vi "Desktop Execution Node - Test Tachometer and Fan Speed IP.vi"() -> ()   [LabVIEW 2014]
uses:
  <vilib>/rvi/DesktopExecutionNode/Execution/niFpgaDEN_Execute.vi
  <vilib>/rvi/DesktopExecutionNode/DesktopExecutionNode.xnode
panel:
  in  "stop":bool
  out "Fan Speed (RPM) Chart":sgl(graph)
  out "Simulated Tachometer Signal":dbl[](graph)
  out "Iteration":i32
  in  "Tach data filename":path=path "Tach - 3000 RPM.tdms"
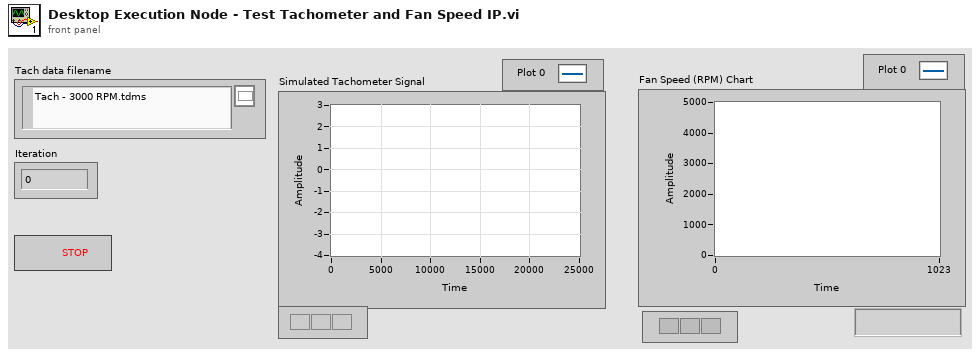
[diagram p1: front panel]
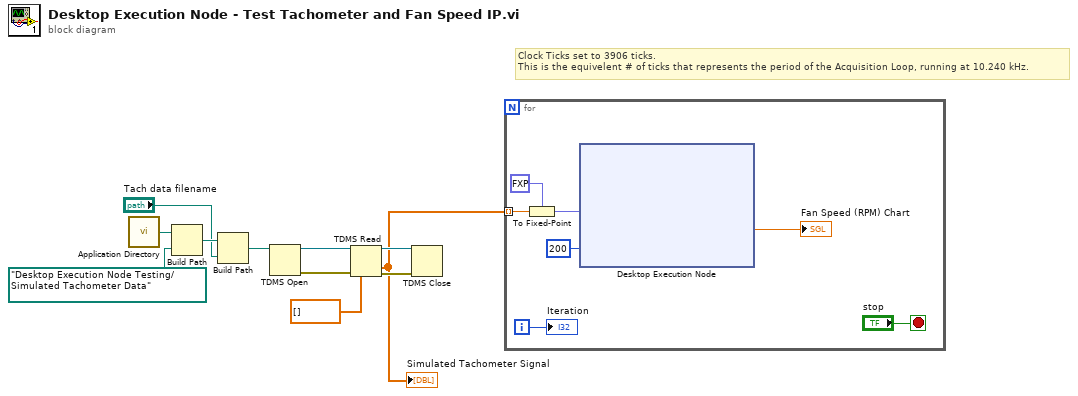
[diagram p0: block diagram]
diagram:
  # "Clock Ticks set to 3906 ticks.\nThis is the equivelent # of ticks that represents the period of the Acquisition Loop, running at 10.240 kHz."
  n1 = call <vilib>:"Application Directory.vi"() -> ("Application Directory"=w5:path)
  n2 = Build Path(base path=w5, name or relative path=path "Desktop Execution Node Testing/Simulated Tachometer Data" ("Application Directory")) -> (appended path=w3:path)
  n3 = Build Path(base path=w3, name or relative path="Tach data filename") -> (appended path=w1:path)
  n4 = TDMS Open(11:w1) -> (0:w10:errorcluster, 3:w11:refnum<k34>)  [unwired: 6 in]
  n5 = TDMS Read(0:w11, 11:w10, 12:dbl[] []) -> (4:w7:refnum<k34>, 10:w6:dbl[], 15:w8:errorcluster)  [unwired: 5 in, 3 out]
  "Simulated Tachometer Signal" <- w6
  n6 = TDMS Close(8:w8, 11:w7) -> ()  [unwired: 2 out]
  n7 = for {
    tunnel: w6 -> [w18] mode=indexing
    i -> [w15]
    stop <- "stop" stop-if-true
    n8 = To Fixed-Point(fixed-point type=fxp<+/-,24,4> 0.0, number=w18) -> (fixed-point=w16:fxp<+/-,24,4>)
    n9 = xnode "Desktop Execution Node"("Tach"=w16, "Requested PID Loop Period (us)"=u32 200) -> ("Fan Speed (RPM)"=→"Fan Speed (RPM) Chart":sgl)  [unwired: 1 in, 1 out]
    "Iteration" <- w15
  }
